vi "Cursors.vi"(1 "Max Jitter Point":cluster{"X":dbl, "Y":dbl}, 2 "standard deviation":dbl, 3 "mean":dbl) -> (0 "Cursor List":T1(array[cluster]))   [LabVIEW 2014]
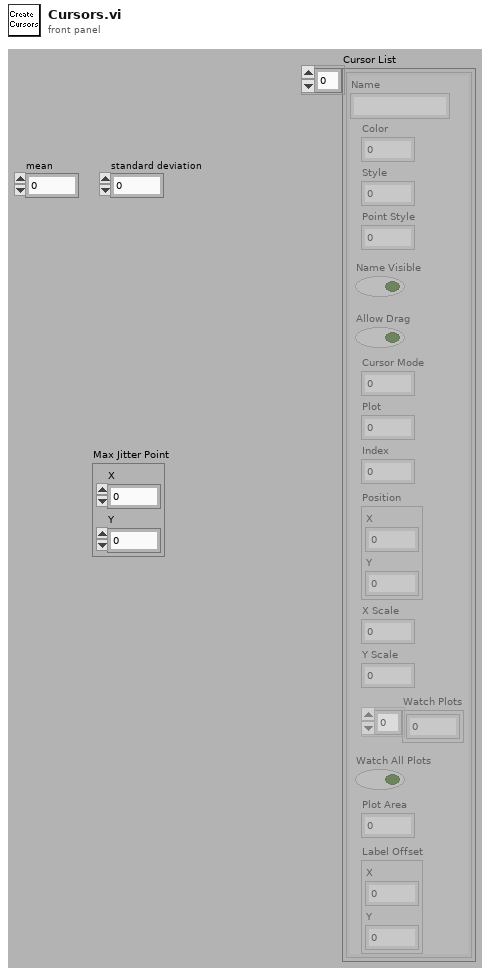
[diagram p1: front panel]
types:
  T1 = cluster{"Name":string, "Color":u32, "Style":u8, "Point Style":u8, "Name Visible":bool, "Allow Drag":bool, "Cursor Mode":u32, "Plot":i32, "Index":i32, "Position":cluster{"X":dbl, "Y":dbl}, "X Scale":u32, "Y Scale":u32, "Watch Plots":i32[], "Watch All Plots":bool, "Plot Area":i32, "Label Offset":cluster{"X":dbl, "Y":dbl}}[]
  T2 = cluster{"Name":string, "Color":u32, "Style":u8, "Point Style":u8, "Name Visible":bool, "Allow Drag":bool, "Cursor Mode":u32, "Plot":i32, "Index":i32, "Position":cluster{"X":dbl, "Y":dbl}, "X Scale":u32, "Y Scale":u32, "Watch Plots":i32[], "Watch All Plots":bool, "Plot Area":i32, "Label Offset":cluster{"X":dbl, "Y":dbl}}
  T3 = cluster{"Cursor Name":string, "Color":u32, "Cursor Style":u8, "Cursor Point Style":u8, "Cursor Name Visible":bool, "Allow Drag":bool, "Cursor Locked":u32, "Cursor Plot":u32, "Cursor Index":i32, cluster{"Cursor X":dbl, "mean":dbl}}
  T4 = cluster{"Cursor Name":string, "Color":u32, "Cursor Style":u8, "Cursor Point Style":u8, "Cursor Name Visible":bool, "Allow Drag":bool, "Cursor Locked":u32, "Cursor Plot":u32, "Cursor Index":i32, cluster{"Cursor X":dbl, dbl}}
  T5 = cluster{"Cursor Name":string, "Color":u32, "Cursor Style":u8, "Cursor Point Style":u8, "Cursor Name Visible":bool, "Allow Drag":bool, "Cursor Locked":u32, "Cursor Plot":u32, "Cursor Index":i32, "Max Jitter Point":cluster{"X":dbl, "Y":dbl}}
  T6 = cluster{"Cursor Name":string, "Color":u32, "Cursor Style":u8, "Cursor Point Style":u8, "Cursor Name Visible":bool, "Allow Drag":bool, "Cursor Locked":u32, "Cursor Plot":u32, "Cursor Index":i32, "Max Jitter Point":cluster{"X":dbl, "Y":dbl}}[]
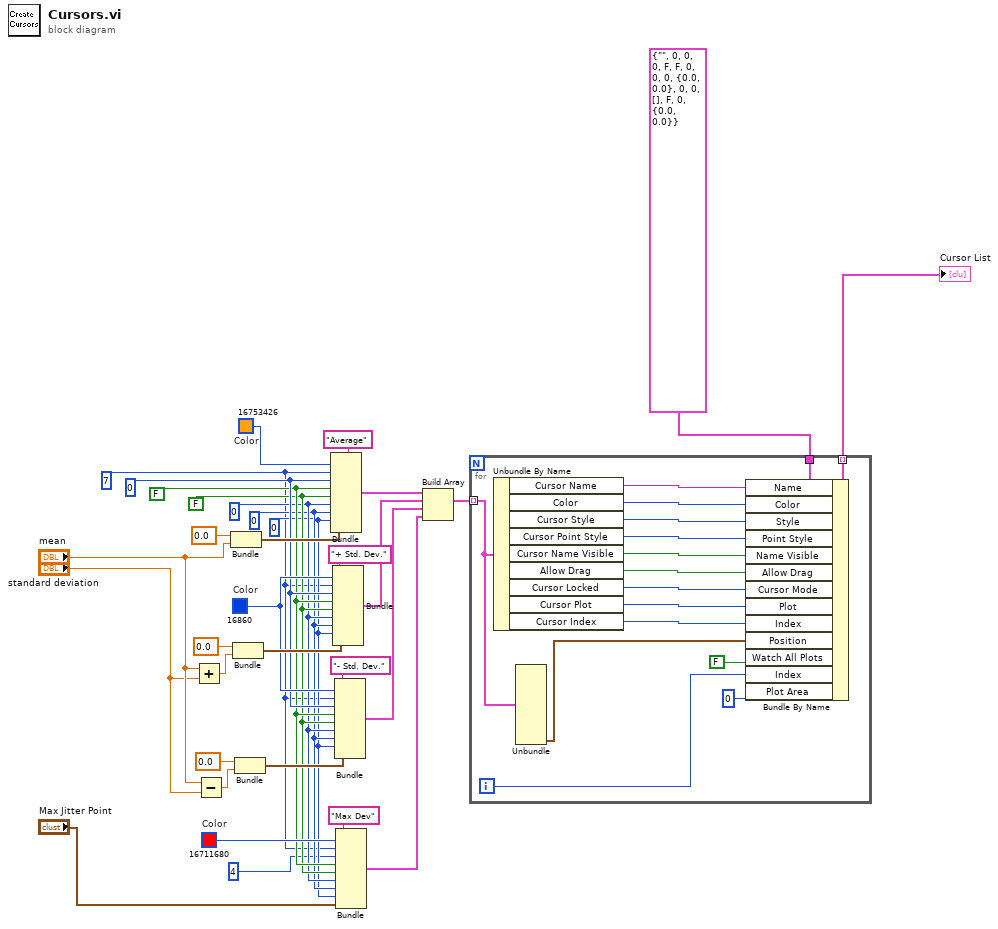
[diagram p0: block diagram]
diagram:
  w11 = u32 16711680  # Color
  w14 = u32 16753426  # Color
  w13 = u32 16860  # Color
  w2 = u8 7 ("Cursor Style")
  w10 = u8 0 ("Cursor Point Style")
  w9 = FALSE ("Cursor Name Visible")
  w8 = FALSE ("Allow Drag")
  w7 = u32 0 ("Cursor Locked")
  w6 = u32 0 ("Cursor Plot")
  w5 = 0 ("Cursor Index")
  n1 = Add(x="mean", y="standard deviation") -> (x+y=w19:dbl)
  n2 = Subtract(x="mean", y="standard deviation") -> (x-y=w18:dbl)
  n3 = Bundle("Cursor X"=0.0, "mean"="mean") -> (w29:cluster{"Cursor X":dbl, "mean":dbl})  [unwired: 1 in]
  n4 = Bundle("Cursor X"=0.0, w19) -> (w27:cluster{"Cursor X":dbl, dbl})  [unwired: 1 in]
  n5 = Bundle("Cursor X"=0.0, w18) -> (w22:cluster{"Cursor X":dbl, dbl})  [unwired: 1 in]
  n6 = Bundle("Cursor Name"="Average", "Color"=w14, "Cursor Style"=w2, "Cursor Point Style"=w10, "Cursor Name Visible"=w9, "Allow Drag"=w8, "Cursor Locked"=w7, "Cursor Plot"=w6, "Cursor Index"=w5, w29) -> (w28:T3)  [unwired: 1 in]
  n7 = Bundle("Cursor Name"="+ Std. Dev.", "Color"=w13, "Cursor Style"=w2, "Cursor Point Style"=w10, "Cursor Name Visible"=w9, "Allow Drag"=w8, "Cursor Locked"=w7, "Cursor Plot"=w6, "Cursor Index"=w5, w27) -> (w21:T4)  [unwired: 1 in]
  n8 = Bundle("Cursor Name"="- Std. Dev.", "Color"=w13, "Cursor Style"=w2, "Cursor Point Style"=w10, "Cursor Name Visible"=w9, "Allow Drag"=w8, "Cursor Locked"=w7, "Cursor Plot"=w6, "Cursor Index"=w5, w22) -> (w20:T4)  [unwired: 1 in]
  n9 = Bundle("Cursor Name"="Max Dev", "Color"=w11, "Cursor Style"=w2, "Cursor Point Style"=u8 4, "Cursor Name Visible"=w9, "Allow Drag"=w8, "Cursor Locked"=w7, "Cursor Plot"=w6, "Cursor Index"=w5, "Max Jitter Point"="Max Jitter Point") -> (w3:T5)  [unwired: 1 in]
  n10 = Build Array(w28, w21, w20, w3) -> (w17:T6)
  n11 = for {
    tunnel: w17 -> [w42] mode=indexing
    tunnel: T2 {"Name"="", "Color"=0, "Style"=0, "Point Style"=0, "Name Visible"=FALSE, "Allow Drag"=FALSE, "Cursor Mode"=0, "Plot"=0, "Index"=0, "Position"={"X"=0.0, "Y"=0.0}, "X Scale"=0, "Y Scale"=0, "Watch Plots"=[], "Watch All Plots"=FALSE, "Plot Area"=0, "Label Offset"={"X"=0.0, "Y"=0.0}} -> [w49]
    tunnel: [w39] -> w16 mode=indexing
    i -> [w37]
    n12 = Unbundle By Name(w42) -> ("Cursor Name"=w48:string, "Color"=w47:u32, "Cursor Style"=w46:u8, "Cursor Point Style"=w45:u8, "Cursor Name Visible"=w44:bool, "Allow Drag"=w43:bool, "Cursor Locked"=w34:u32, "Cursor Plot"=w35:u32, "Cursor Index"=w40:i32)
    n13 = Unbundle(w42) -> ("Max Jitter Point"=w41:cluster{"X":dbl, "Y":dbl})  [unwired: 9 out]
    n14 = Bundle By Name(cluster=w49, "Name"=w48, "Color"=w47, "Style"=w46, "Point Style"=w45, "Name Visible"=w44, "Allow Drag"=w43, "Cursor Mode"=w34, "Plot"=w35, "Index"=w40, "Position"=w41, "Watch All Plots"=FALSE, "Index"=w37, "Plot Area"=0) -> (w39:T2)
  }
  "Cursor List" <- w16
